vi "Cook Current Recipe Step.vi"(8 "error in (no error)":errorcluster, 11 "Cooker Actor in":refnum<class "Cooker Actor.lvclass">) -> (0 "error out":errorcluster, 3 "Cooker Actor out":refnum<class "Cooker Actor.lvclass">)   [LabVIEW 2024, in "Cooker Actor.lvlib" / "Cooker Actor.lvclass"]
uses:
  Cooker Actor.lvclass
  Cooker Actor.lvclass/Cooker Actor.ctl
  Oven Actor/Oven Actor Messages/Apply Heat Msg/Apply Heat Msg.lvclass
  Timer Actor/Timer Actor Messages/Start Count Down Msg/Start Count Down Msg.lvclass
  Recipe Actor/Recipe Step/Recipe Step.lvclass
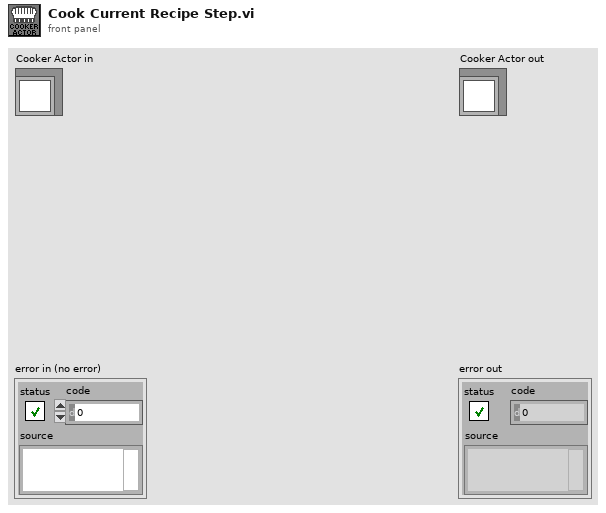
[diagram p1: front panel]
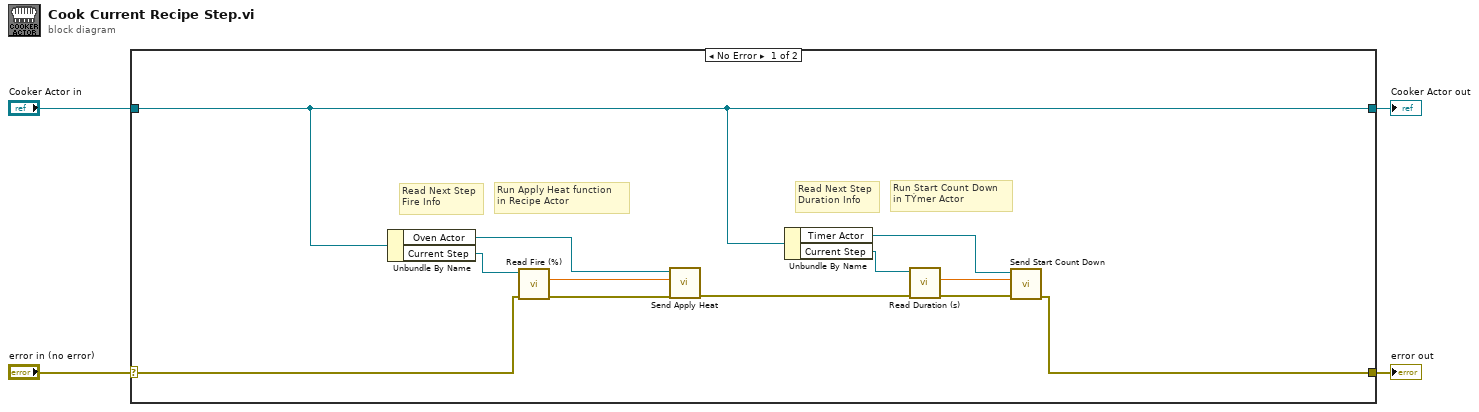
[diagram p0: block diagram]
diagram:
  n1 = case shown="No Error" "error in (no error)" {
    selector: "error in (no error)" -> [w6 w18]
    tunnel: [w5 w18] -> w3
    tunnel: [w7 w17] -> w1
    tunnel: "Cooker Actor in" -> [w7 w17]
    frame No Error {
      # "Run Start Count Down\nin TÝmer Actor"
      # "Read Next Step\nDuration Info"
      # "Run Apply Heat function\nin Recipe Actor"
      # "Read Next Step\nFire Info"
      n2 = Unbundle By Name(w7) -> ("Oven Actor"=w13:refnum<class "Message Enqueuer.lvclass">, "Current Step"=w16:refnum<class "Recipe Step.lvclass">)
      n3 = call-dynamic "Read Fire (%).vi"("error in (no error)"=w6, "Recipe Step in"=w16) -> ("error out"=w14:errorcluster, "Fire (%)"=w15:dbl)  [unwired: 7 in, 1 out]
      n4 = call "Send Apply Heat.vi"("error in (no error)"=w14, "Fire (%)"=w15, "Message Enqueuer"=w13) -> ("error out"=w12:errorcluster)  [unwired: 7 in, 1 out]
      n5 = Unbundle By Name(w7) -> ("Timer Actor"=w8:refnum<class "Message Enqueuer.lvclass">, "Current Step"=w11:refnum<class "Recipe Step.lvclass">)
      n6 = call-dynamic "Read Duration (s).vi"("error in (no error)"=w12, "Recipe Step in"=w11) -> ("error out"=w10:errorcluster, "Duration (s)"=w9:dbl)  [unwired: 7 in, 1 out]
      n7 = call "Send Start Count Down.vi"("error in (no error)"=w10, "Seconds To Wait"=w9, "Message Enqueuer"=w8) -> ("error out"=w5:errorcluster)  [unwired: 7 in, 1 out]
    }
    frame Error {
    }
  }
  "error out" <- w3
  "Cooker Actor out" <- w1
